vi "hmi_swap_monitor.vi"(8 "error in (no error)":errorcluster, 10 "callee_vi_refnum":refnum<vi>, 11 "caller_vi_refnum":refnum<vi>) -> (0 "error out":errorcluster)   [LabVIEW 2015, in "lv-dialog-interfaces.lvlib"]
uses:
  lv-dialog-interfaces.lvlib
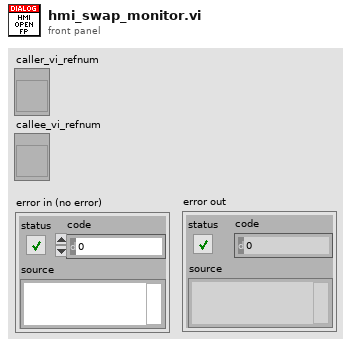
[diagram p1: front panel]
types:
  T1 = enum32{"Invalid", "Standard", "Closed", "Hidden", "Minimized", "Maximized"}
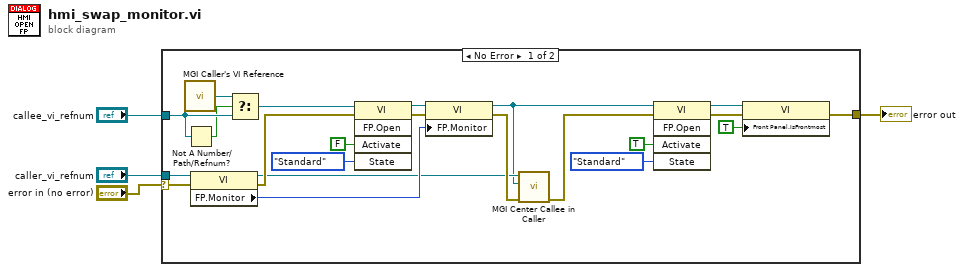
[diagram p0: block diagram]
diagram:
  n1 = case shown="No Error" "error in (no error)" {
    selector: "error in (no error)" -> [w25 w27]
    tunnel: [w9 w27] -> w4
    tunnel: "callee_vi_refnum" -> [w8 _]
    tunnel: "caller_vi_refnum" -> [w26 _]
    frame No Error {
      n2 = call "MGI Caller's VI Reference.vi"() -> ("Caller's VI Reference"=w5:refnum<vi>)  [unwired: 1 in]
      n3 = Not A Number/Path/Refnum?(number/path/refnum=w8) -> (NaN/Path/Refnum?=w6:bool)
      n4 = property class="VI"(reference=w26, error in=w25) -> (reference out=w21:refnum<vi>, error out=w24:errorcluster, "FP.Monitor"=w23:u16)
      n5 = Select(t=w5, s=w6, f=w8) -> (s? t:f=w7:refnum<vi>)
      n6 = invoke class="VI" method="FP.Open"(reference=w7, error in=w24, "Activate"=FALSE ("Activate?"), "State"=T1."Standard") -> (reference out=w14:refnum<vi>, error out=w13:errorcluster)  [unwired: 1 in, 3 out]
      n7 = property class="VI"(reference=w14, error in=w13, "FP.Monitor"=w23) -> (reference out=w18:refnum<vi>, error out=w22:errorcluster)
      n8 = call "MGI Center Callee in Caller.vi"("Error In"=w22, "Callee VI Refnum (Caller)"=w18, "Caller VI Refnum (Callee's Caller)"=w21) -> ("Error Out"=w17:errorcluster)  [unwired: 8 in]
      n9 = invoke class="VI" method="FP.Open"(reference=w18, error in=w17, "Activate"=TRUE ("Activate?"), "State"=T1."Standard") -> (reference out=w12:refnum<vi>, error out=w11:errorcluster)  [unwired: 1 in, 3 out]
      n10 = property class="VI"(reference=w12, error in=w11, "Front Panel.IsFrontmost"=TRUE ("Front Panel Window:Is Frontmost")) -> (error out=w9:errorcluster)  [unwired: 1 out]
    }
    frame Error {
    }
  }
  "error out" <- w4
